vi "test.vi"() -> ()   [LabVIEW 2018]
panel:
  in  "File Information":T1
  in  "stop":bool
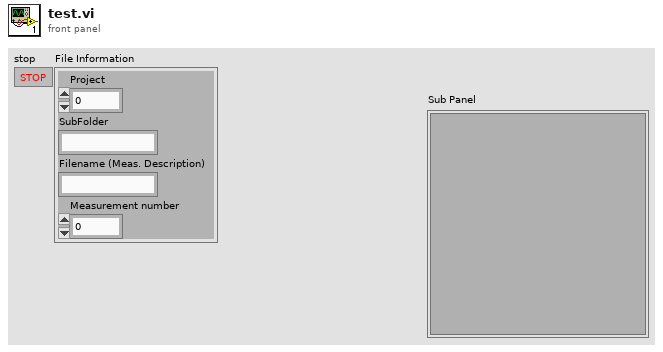
[diagram p1: front panel]
types:
  T1 = cluster{"Project":u16, "SubFolder":string, "Filename (Meas. Description)":string, "Measurement number":i32}
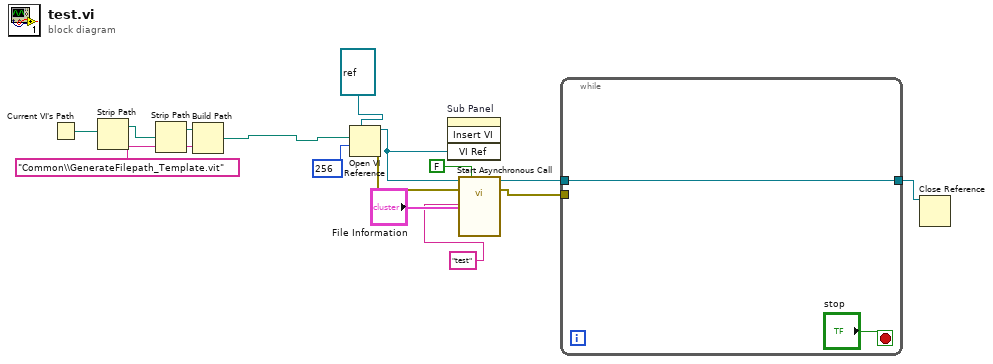
[diagram p0: block diagram]
diagram:
  n1 = Current VI's Path() -> (path=w10:path)
  n2 = Strip Path(path=w10) -> (stripped path=w9:path)  [unwired: 1 out]
  n3 = Strip Path(path=w9) -> (stripped path=w12:path)  [unwired: 1 out]
  n4 = Build Path(base path=w12, name or relative path="Common\\GenerateFilepath_Template.vit") -> (appended path=w8:path)
  n5 = Open VI Reference(type specifier VI Refnum (for type only)=refnum<vi> refnum, vi path=w8, options=256) -> (vi reference=w15:refnum<vi>, error out=w14:errorcluster)  [unwired: 1 in, 2 out]
  n6 = invoke on="Sub Panel" class="SubPnl" method="Insert VI"("VI Ref"=w15) -> ()  [unwired: 3 in, 4 out]
  n7 = call-by-ref "Start Asynchronous Call"(reference=w15, error in=w14, "Check for file?"=FALSE, "File Information"="File Information", "Instrument"="test") -> (reference out=w6:refnum<vi>, error out=w5:errorcluster)  [unwired: 3 out]
  n8 = while {
    tunnel: w6 -> [w16]
    tunnel: w5 -> [_]
    tunnel: [w16] -> w1
    stop <- "stop" stop-if-true
  }
  n9 = Close Reference(reference=w1) -> ()  [unwired: 1 in, 1 out]
